vi "do get loop iteration terminal.vi"(8 "error in (no error)":errorcluster, 10 "get_loop_iteration_terminal Argument":T3, 11 "Data Cluster in":T1) -> (0 "error out":errorcluster, 2 "get_loop_iteration_terminal (Reply Payload)":T2, 3 "Data Cluster out":T1)   [LabVIEW 2025, in "Scripting Server.lvlib"]
uses:
  Scripting Server.lvlib
  get_loop_iteration_terminal (Reply Payload)--cluster.ctl
  Module Data--cluster.ctl
  get_loop_iteration_terminal Argument--cluster.ctl
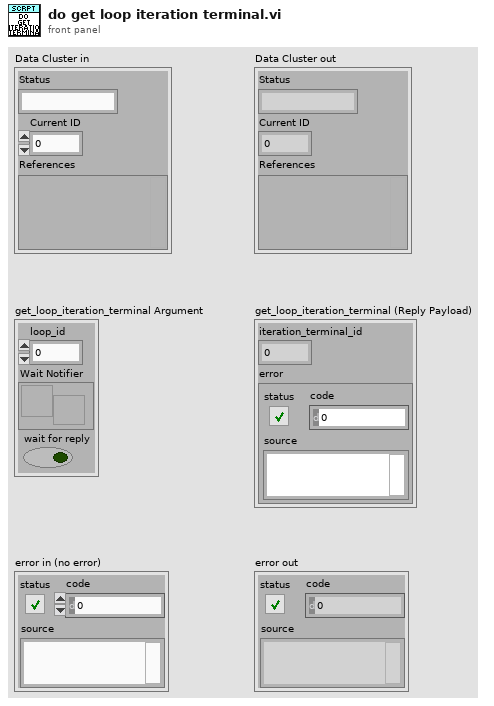
[diagram p1: front panel]
types:
  T1 = typedef "Scripting Server.lvlib/Module Data--cluster.ctl" = cluster{"Status":string, "Current ID":i32, "References":variant}
  T2 = typedef "Scripting Server.lvlib/get_loop_iteration_terminal (Reply Payload)--cluster.ctl" = cluster{"iteration_terminal_id":i32, "error":errorcluster}
  T3 = typedef "Scripting Server.lvlib/get_loop_iteration_terminal Argument--cluster.ctl" = cluster{"loop_id":i32, "Wait Notifier":refnum<notifier>, "wait for reply":bool}
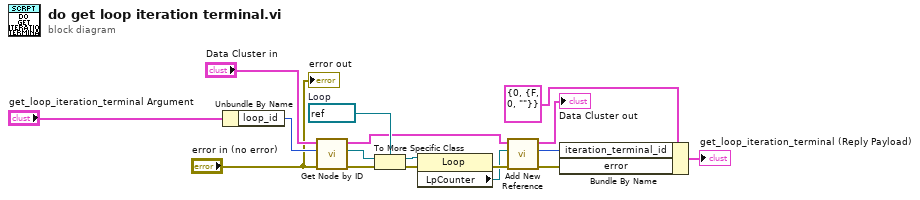
[diagram p0: block diagram]
diagram:
  w9 = refnum<vi> refnum  # Loop
  n1 = Unbundle By Name("get_loop_iteration_terminal Argument") -> ("loop_id"=w12:i32)
  n2 = call "Get Node by ID.vi"("error in (no error)"="error in (no error)", "ID"=w12, "Data Cluster in"="Data Cluster in") -> ("error out"=w14:errorcluster, "specific class reference"=w10:refnum<vi>, "Data Cluster out"=w6:T1)  [unwired: 6 in]
  n3 = To More Specific Class(target class=w9, reference=w10, error in=w14) -> (specific class reference=w7:refnum<vi>, error out=w11:errorcluster)
  n4 = property class="Loop"(reference=w7, error in=w11) -> (error out=w8:errorcluster, "LpCounter"=w4:refnum<vi>)  [unwired: 1 out]
  n5 = call "Add New Reference.vi"("error in (no error)"=w8, "Variant"=w4, "Data Cluster in"=w6) -> ("error out"=w2:errorcluster, "new reference"=w3:i32, "Data Cluster out 2"=→"Data Cluster out":T1)  [unwired: 6 in]
  n6 = Bundle By Name(cluster=T2 {"iteration_terminal_id"=0, "error"={"status"=FALSE, "code"=0, "source"=""}} ("get_loop_iteration_terminal (Reply Payload)"), "iteration_terminal_id"=w3, "error"=w2) -> (→"get_loop_iteration_terminal (Reply Payload)":T2)
  "error out" <- "error in (no error)"
